vi "GreenQuotes.vi"(11 "String in":refnum<vi>) -> (3 "String out":refnum<vi>)   [LabVIEW 2020]
uses:
  ColorGlobals.vi
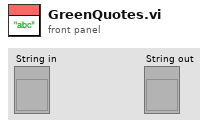
[diagram p1: front panel]
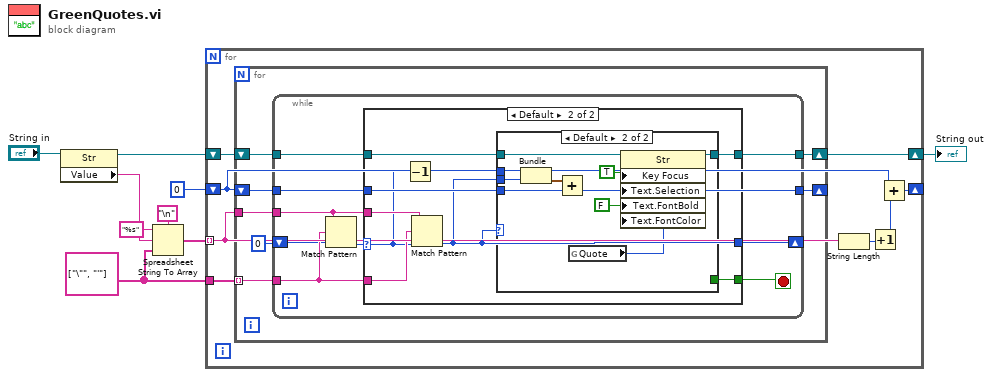
[diagram p0: block diagram]
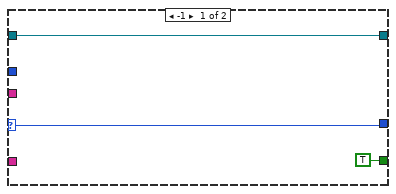
[diagram p2: hidden frame]
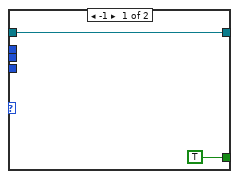
[diagram p3: hidden frame]
diagram:
  w8 = string[] ["\"", "'"]
  n1 = property on="Property Node" class="Str"(reference="String in") -> (reference out=w2:refnum<vi>, "Value"=w3:string)  [unwired: 1 in, 1 out]
  n2 = Spreadsheet String To Array(delimiter (Tab)="\n", format string="%s", spreadsheet string=w3, array type (2D Dbl)=w8) -> (array=w7:string[])
  n3 = for {
    tunnel: w8 -> [w16]
    shift-right: [w15] -> w1
    shift-left: w2 -> [w17]
    tunnel: w7 -> [w10] mode=indexing
    shift-right: [w13] -> _
    shift-left: 0 -> [w12]
    n4 = for {
      tunnel: w10 -> [w21]
      tunnel: w16 -> [w22] mode=indexing
      shift-right: [w23] -> w15
      shift-left: w17 -> [w24]
      shift-right: [w19] -> _
      shift-left: w12 -> [w20]
      n5 = while {
        tunnel: w21 -> [w31]
        shift-right: [w33] -> _
        shift-left: 0 -> [w25]
        tunnel: w24 -> [w32]
        tunnel: [w30] -> w23
        tunnel: w22 -> [w28]
        tunnel: w20 -> [w26]
        tunnel: [w26] -> w19
        stop <- w29 stop-if-true
        n6 = Match Pattern(string=w31, regular expression=w28, offset (0)=w25) -> (offset past match=w27:i32)  [unwired: 3 out]
        n7 = case shown="Default" w27 {
          selector: w27 -> [w35 w39]
          tunnel: [w35 w42] -> w33
          tunnel: w32 -> [w36 w45]
          tunnel: w31 -> [_ w44]
          tunnel: [w36 w43] -> w30
          tunnel: [TRUE w41] -> w29
          tunnel: w28 -> [_ w40]
          tunnel: w26 -> [_ w38]
          frame -1 {
          }
          frame Default {
            n8 = Decrement(x=w39) -> (x-1=w37:i32)
            n9 = Match Pattern(string=w44, regular expression=w40, offset (0)=w39) -> (offset past match=w42:i32)  [unwired: 3 out]
            n10 = case shown="Default" w42 {
              tunnel: w42 -> [_ w57]
              tunnel: w45 -> [w46 w54]
              tunnel: [w46 w53] -> w43
              tunnel: [TRUE _] -> w41
              tunnel: w37 -> [_ w52]
              tunnel: w38 -> [_ w49]
              frame -1 {
              }
              frame Default {
                n11 = Bundle(w52, "offset past match"=w57) -> (w51:cluster{i32, "offset past match":i32})  [unwired: 1 in]
                n12 = Add(x=w51, y=w49) -> (x+y=w50:cluster{i32, "offset past match":i32})
                n13 = global read "ColorGlobals.vi" "Quote"() -> (w48:u32)
                n14 = property on="Property Node" class="Str"(reference=w54, "Key Focus"=TRUE, "Text.Selection"=w50, "Text.FontBold"=FALSE ("Text.Font:Bold"), "Text.FontColor"=w48) -> (reference out=w53:refnum<vi>)  [unwired: 1 in, 1 out]
              }
            }
          }
        }
      }
    }
    n15 = String Length(string=w10) -> (length=w14:i32)
    n16 = Increment(x=w14) -> (x+1=w11:i32)
    n17 = Add(x=w12, y=w11) -> (x+y=w13:i32)
  }
  "String out" <- w1
